vi "Read Cnfg File.vi"(0 "Config File":path, 11 "error in (no error)":errorcluster) -> (4 "Last Change":timestamp, 6 "InstalledDGs":T12[](array[typedef]), 8 "DGSystems":T13[](array[typedef]), 10 "Cards":T6[](array[typedef]) {"Advanced Settings"."Trigger on MS Bus" format="%04x" items=["Local Primary0x1"=1, "Local Secondary0x2"=2, "Local Force 0x4"=4, "Resynchronize 0x8"=8, "StepBackOnBus 0x10"=16, "StartOnBus 0x20"=32, "InhibitOnBus 0x40"=64, "LoadDataOnBus 0x80"=128]; "Advanced Settings"."Force Trigger (µs)" min=0.0 format="%.6f"; "SG08_Settings"."StepBackTime (µs)" min=0.0 format="%.6f"; "SG08_Settings"."Gate Delay (µs)" format="%.3f"; "SG08_Settings"."Gate Level" min=-2.5 max=2.5 format="%.3g"; "Base Settings"."Gate Divider" min=1 max=1000000; "Base Settings"."Clock Source" items=["Internal Oscillator"=1, "External Trigger"=2, "Trigger-> Oscillator"=3, "MasterSlave Bus"=4]; "Base Settings"."Inhibit(µs)" format="%#_11g"}, 14 "Chnls":T1[](array[typedef]) {"ChnParameter"."Delay (µs)" min=0.0 max=100000000.0 format="%.4f"; "G08_Chnl_Settings"."Pulse Width (µs)" min=0.0 max=8947840.0 format="%#.6f"; "Go and Done Signal"."Done Signal" format="%04x" items=["Local Primary"=1, "Local Secondary"=2, "Local Force"=4, "Master Primary"=16]; "Go and Done Signal"."Go Signal" format="%04x" items=["Local Primary0x1"=1, "Local Secondary0x2"=2, "Local Force 0x4"=4, "Resynchronize 0x8"=8, "Master Prim. 0x10"=16, "Master Sec. 0x20"=32, "Master Force  0x40"=64, "System Clock 0x80"=128, "Delay Clock 0x100"=256, "Inhibit Local 0x200"=512, "Start Local 0x400"=1024, "Start Bus 0x800"=2048, "Step Back Local 0x1000"=4096, "Step Back Bus 0x2000"=8192, "RunCircle 0x4000"=16384, "SyncReload 0x8000"=32768, "From E 0x10000"=65536, "From F 0x20000"=131072, "From Bus 0x40000"=262144]}, 15 "error out":errorcluster)   [LabVIEW 2009, in "POLARIS BME DG.lvlib" / "BME_DG_System.lvclass"]
uses:
  BME_DG_System.lvclass
  DetectDG.ctl
  System DG Selection.ctl
  Card Config.ctl
  LV-BME Interface/BME_DG_TriggerSettings.ctl
  LV-BME Interface/ClockSource.ctl
  SG08_Settings.ctl
  LV-BME Interface/BME_DG_V2TriggerSettings.ctl
  MSBusSignals.ctl
  Chnl Settings Complete.ctl
  LV-BME Interface/ChnlSettings.ctl
  Go_Done_Chnl_Settings.ctl
  GoSignalBits.ctl
  SG08_Chnl_Settings.ctl
  <vilib>/Utility/xml.llb/Read From XML File(array).vi
  POLARIS BME DG.lvlib
panel:
  in  "Chnls":T1[](array[typedef]) {"ChnParameter"."Delay (µs)" min=0.0 max=100000000.0 format="%.4f"; "G08_Chnl_Settings"."Pulse Width (µs)" min=0.0 max=8947840.0 format="%#.6f"; "Go and Done Signal"."Done Signal" format="%04x" items=["Local Primary"=1, "Local Secondary"=2, "Local Force"=4, "Master Primary"=16]; "Go and Done Signal"."Go Signal" format="%04x" items=["Local Primary0x1"=1, "Local Secondary0x2"=2, "Local Force 0x4"=4, "Resynchronize 0x8"=8, "Master Prim. 0x10"=16, "Master Sec. 0x20"=32, "Master Force  0x40"=64, "System Clock 0x80"=128, "Delay Clock 0x100"=256, "Inhibit Local 0x200"=512, "Start Local 0x400"=1024, "Start Bus 0x800"=2048, "Step Back Local 0x1000"=4096, "Step Back Bus 0x2000"=8192, "RunCircle 0x4000"=16384, "SyncReload 0x8000"=32768, "From E 0x10000"=65536, "From F 0x20000"=131072, "From Bus 0x40000"=262144]}
  in  "Card Config":T6[](array[typedef]) {"Advanced Settings"."Trigger on MS Bus" format="%04x" items=["Local Primary0x1"=1, "Local Secondary0x2"=2, "Local Force 0x4"=4, "Resynchronize 0x8"=8, "StepBackOnBus 0x10"=16, "StartOnBus 0x20"=32, "InhibitOnBus 0x40"=64, "LoadDataOnBus 0x80"=128]; "Advanced Settings"."Force Trigger (µs)" min=0.0 format="%.6f"; "SG08_Settings"."StepBackTime (µs)" min=0.0 format="%.6f"; "SG08_Settings"."Gate Delay (µs)" format="%.3f"; "SG08_Settings"."Gate Level" min=-2.5 max=2.5 format="%.3g"; "Base Settings"."Gate Divider" min=1 max=1000000; "Base Settings"."Clock Source" items=["Internal Oscillator"=1, "External Trigger"=2, "Trigger-> Oscillator"=3, "MasterSlave Bus"=4]; "Base Settings"."Inhibit(µs)" format="%#_11g"}
  in  "Systems 2":T13[](array[typedef])
  in  "InstalledDGs 2":T12[](array[typedef])
  in  "Last Change 2":timestamp
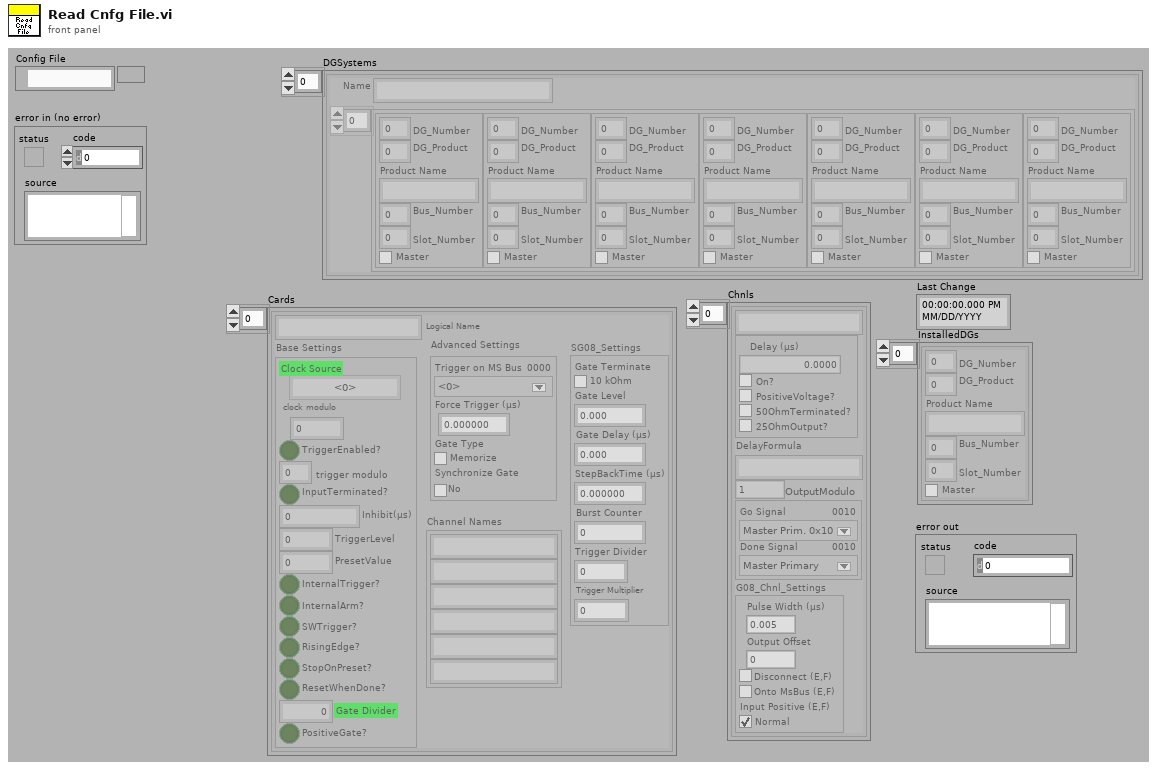
[diagram p1: front panel]
types:
  T1 = typedef "POLARIS BME DG.lvlib/Chnl Settings Complete.ctl" = cluster{"Channel Name":string, "ChnParameter":T2, "DelayFormula":string, "OutputModulo":i32, "Go and Done Signal":T3, "G08_Chnl_Settings":T5}
  T2 = typedef "POLARIS BME DG.lvlib/ChnlSettings.ctl" = cluster{" Delay (µs)":dbl, "On?":bool, "PositiveVoltage?":bool, "50OhmTerminated? ":bool, "25OhmOutput?":bool}
  T3 = typedef "POLARIS BME DG.lvlib/Go_Done_Chnl_Settings.ctl" = cluster{"Go Signal":T4, "Done Signal":u32}
  T4 = typedef "POLARIS BME DG.lvlib/GoSignalBits.ctl" = u32
  T5 = typedef "POLARIS BME DG.lvlib/SG08_Chnl_Settings.ctl" = cluster{"Pulse Width (µs)":dbl, "Output Offset":u32, "Disconnect (E,F)":bool, "Onto MsBus (E,F)":bool, "Input Positive (E,F)":bool}
  T6 = typedef "POLARIS BME DG.lvlib/Card Config.ctl" = cluster{"Logical Name":string, "Base Settings":T7, "SG08_Settings":T9, "Channel Names":string[], "Advanced Settings":T10}
  T7 = typedef "POLARIS BME DG.lvlib/BME_DG_TriggerSettings.ctl" = cluster{"Clock Source":T8, " clock modulo":u32, "TriggerEnabled?":bool, "trigger modulo ":i32, "InputTerminated?":bool, "Inhibit(µs)":dbl, "TriggerLevel":dbl, "PresetValue":i32, "InternalTrigger?":bool, "InternalArm?":bool, "SWTrigger?":bool, "RisingEdge?":bool, "StopOnPreset?":bool, "ResetWhenDone?":bool, "Gate Divider":i32, "PositiveGate?":bool}
  T8 = typedef "POLARIS BME DG.lvlib/ClockSource.ctl" = i32
  T9 = typedef "POLARIS BME DG.lvlib/SG08_Settings.ctl" = cluster{"Gate Terminate":bool, "Gate Level":dbl, "Gate Delay (µs)":dbl, "StepBackTime (µs)":dbl, "Burst Counter":u32, "Trigger Divider":u32, "Trigger Multiplier":u32}
  T10 = typedef "POLARIS BME DG.lvlib/BME_DG_V2TriggerSettings.ctl" = cluster{"Trigger on MS Bus":T11, "Force Trigger (µs)":dbl, "Gate Type":bool, "Synchronize Gate":bool}
  T11 = typedef "POLARIS BME DG.lvlib/MSBusSignals.ctl" = u32
  T12 = typedef "POLARIS BME DG.lvlib/DetectDG.ctl" = cluster{"DG_Number":i32, "DG_Product":i32, "Product Name":string, "Bus_Number":i32, "Slot_Number":i32, "Master":bool}
  T13 = typedef "POLARIS BME DG.lvlib/System DG Selection.ctl" = cluster{"Selected System DGs":T12[], "Name":string}
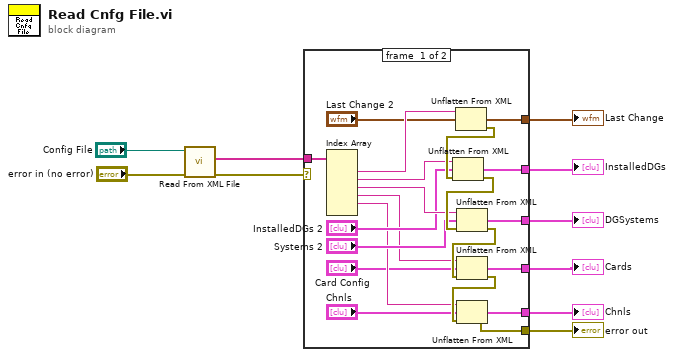
[diagram p0: block diagram]
diagram:
  n1 = call-poly <vilib>:"Read From XML File.vi"("error in (no error)"="error in (no error)", "XML File Path"="Config File") -> ("error out"=w5:errorcluster, "XML Elements"=w6:string[])  [unwired: 7 in, 1 out]
  n2 = case shown="No Error" w5 {
    selector: w5 -> [_ w32]
    tunnel: w6 -> [w31 _]
    tunnel: [w28 _] -> w7
    tunnel: [w22 _] -> w8
    tunnel: [w21 _] -> w10
    tunnel: [w18 w32] -> w9
    tunnel: [w12 _] -> w2
    tunnel: [w11 _] -> w1
    frame #0 {
      n3 = Index Array(array=w31) -> (element #1=w30:string, element #2=w13:string, element #3=w25:string, element #4=w17:string, element #5=w16:string)  [unwired: 6 in, 1 out]
      n4 = Unflatten From XML(xml string=w30, type="Last Change 2") -> (value=w28:timestamp, error out=w27:errorcluster)  [unwired: 1 in]
      n5 = Unflatten From XML(xml string=w13, type="InstalledDGs 2", error in (no error)=w27) -> (value=w22:T12[], error out=w26:errorcluster)
      n6 = Unflatten From XML(xml string=w25, type="Systems 2", error in (no error)=w26) -> (value=w21:T13[], error out=w20:errorcluster)
      n7 = Unflatten From XML(xml string=w17, type="Card Config", error in (no error)=w20) -> (value=w12:T6[], error out=w19:errorcluster)
      n8 = Unflatten From XML(xml string=w16, type="Chnls", error in (no error)=w19) -> (value=w11:T1[], error out=w18:errorcluster)
    }
    frame #1 {
    }
  }
  "DGSystems" <- w10
  "error out" <- w9
  "InstalledDGs" <- w8
  "Last Change" <- w7
  "Cards" <- w2
  "Chnls" <- w1
